vi "Get Bookmarks Map.vi"(8 "error in (no error)":errorcluster {"code" format="Error %.0f"}, 11 "VIDoc Parser in":refnum<class "VIDoc Parser.lvclass">) -> (0 "error out":errorcluster {"code" format="Error %.0f"}, 2 "Bookmarks to Term Map":map{string, string}(c390), 3 "VIDoc Parser out":refnum<class "VIDoc Parser.lvclass">)   [LabVIEW 2023, in "VIDoc Parsing.lvlib" / "VIDoc Parser.lvclass"]
uses:
  VIDoc Parser.lvclass
  VIDoc Parser.lvclass/VIDoc Parser.ctl
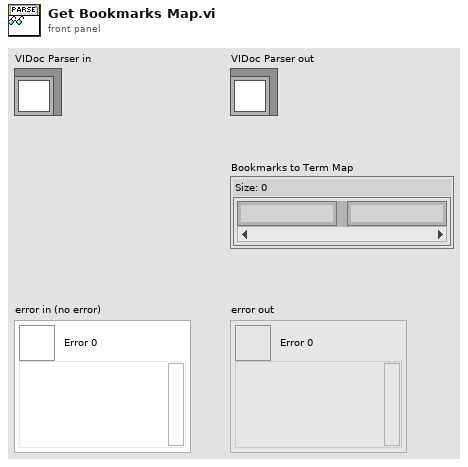
[diagram p1: front panel]
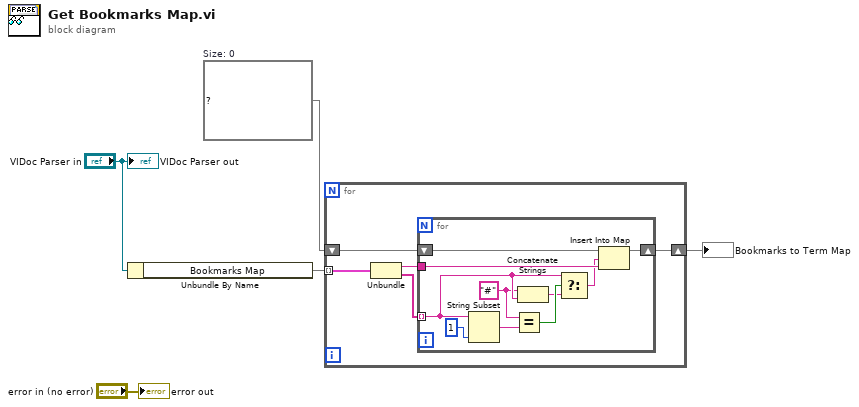
[diagram p0: block diagram]
diagram:
  w2 = map{string, string} {}  # Size: 0
  n1 = Unbundle By Name("VIDoc Parser in") -> ("Bookmarks Map"=w3:map{string, string[]})
  n2 = for {
    tunnel: w3 -> [w10] mode=indexing
    shift-right: [w8] -> w1
    shift-left: w2 -> [w9]
    n3 = Unbundle(w10) -> ("Term"=w6:string, "Bookmarks"=w7:string[])
    n4 = for {
      tunnel: w7 -> [w14] mode=indexing
      shift-right: [w19] -> w8
      shift-left: w9 -> [w20]
      tunnel: w6 -> [w18]
      w13 = "#" ("x")
      n5 = String Subset(string=w14, length (rest)=1 ("length (rest)")) -> (substring=w16:string)  [unwired: 1 in]
      n6 = Equal?(x=w13, y=w16) -> (x = y?=w15:bool)
      n7 = Concatenate Strings(w13, w14) -> (w12:string)
      n8 = Select(t=w14, s=w15, f=w12) -> (s? t:f=w11:string)
      n9 = Insert Into Map(map in=w20, key=w11, value=w18) -> (map out=w19:map{string, string})  [unwired: 2 out]
    }
  }
  "Bookmarks to Term Map" <- w1
  "error out" <- "error in (no error)"
  "VIDoc Parser out" <- "VIDoc Parser in"
